vi "GetSetAccessLevel.vi"(8 "error in":errorcluster, 9 "Access level":u8 max=5 step=1, 10 "get/set":T1, 11 "VISA resource name":refnum<visa-resource-name>) -> (0 "error out":errorcluster, 2 "Access level response":string, 3 "VISA resource name out":refnum<visa-resource-name>)   [LabVIEW 2023, in "Thermotron 8800.lvlib"]
doc: "LOCK\nCommand name: Send or load access level\nCommand type: System status\nDescription: This is the only system status command that allows you to change the 8800’s status. It allows you to read and change the access level of the 8800.\nSyntax: LOCK? or LOCKn\nWhere n indicates access level (0 through 5):\n0 Locked 3 Programmer 1 Level One 4 Lab Manager 2 Level Two 5 Calibration\nData type: Coded integer\nQuery example: LOCK?\n8800 response: 3 (The 8800 is set to the Programmer access level.)\nOperation example: LOCK0\n8800 response: This command locks out all user access to the 8800 functions at the keyboard."
uses:
  Thermotron 8800.lvlib
  Private/get set.ctl
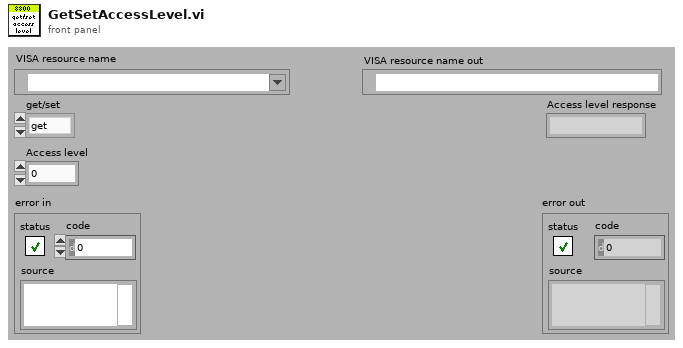
[diagram p1: front panel]
types:
  T1 = typedef "Thermotron 8800.lvlib/get set.ctl" = enum16{"get", "set"}
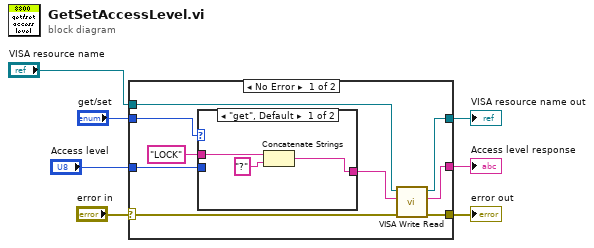
[diagram p0: block diagram]
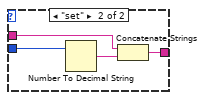
[diagram p2: hidden frame]
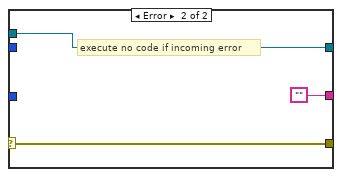
[diagram p3: hidden frame]
diagram:
  n1 = case shown="No Error" "error in" {
    selector: "error in" -> [w8 w25]
    tunnel: "get/set" -> [w16 _]
    tunnel: [w13 ""] -> w1
    tunnel: [w12 w25] -> w5
    tunnel: [w11 w26] -> w4
    tunnel: "VISA resource name" -> [w10 w26]
    tunnel: "Access level" -> [w9 _]
    frame No Error {
      n2 = case shown="\"get\", Default" w16 {
        tunnel: "LOCK" ("8800 Command") -> [w18 w23]
        tunnel: [w19 w22] -> w14
        tunnel: w9 -> [_ w20]
        frame "get", Default {
          n3 = Concatenate Strings(w18, "?" ("8800 Command")) -> (w19:string)
        }
        frame "set" {
          n4 = Number To Decimal String(number=w20) -> (decimal integer string=w21:string)  [unwired: 1 in]
          n5 = Concatenate Strings(w23, w21) -> (w22:string)
        }
      }
      n6 = call "VISA Write Read.vi"("error in (no error)"=w8, "8800 Command"=w14, "VISA Refnum in"=w10) -> ("error out"=w12:errorcluster, "read buffer"=w13:string, "VISA Refnum out"=w11:refnum<visa-resource-name>)  [unwired: 6 in]
    }
    frame Error {
      # "execute no code if incoming error"
    }
  }
  "VISA resource name out" <- w4
  "error out" <- w5
  "Access level response" <- w1
